vi "Close.vi"(8 "error in (no error)":errorcluster, 11 "Sequence Call Step Dict in":refnum<class "Sequence Call Step Dictionary.lvclass">) -> (0 "error out":errorcluster)   [LabVIEW 2018, in "Sequence Call Step Dictionary.lvlib" / "Sequence Call Step Dictionary.lvclass"]
uses:
  Sequence Call Step Dictionary.lvclass
  Sequence Call Step Dictionary.lvclass/Sequence Call Step Dictionary.ctl
  Controls/Sequence Call Step.ctl
  Controls/Parameter.ctl
  Private Methods/Read Database.vi
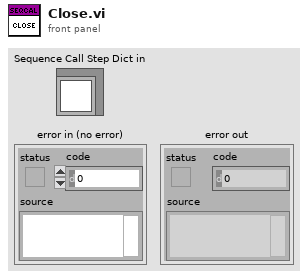
[diagram p1: front panel]
types:
  T1 = typedef "Sequence Call Step Dictionary.lvlib/Sequence Call Step Dictionary.lvclass/Sequence Call Step.ctl" = cluster{"Sequence Call Step Reference":refnum<k7>, "Sequence Call Parameters":T2[]}
  T2 = typedef "Sequence Call Step Dictionary.lvlib/Sequence Call Step Dictionary.lvclass/Parameter.ctl" = cluster{"Name":string, "PropertyObject Type":enum16{"Container", "String", "Boolean", "Number", "NamedType", "Reference", "Array", "Aperture Time"}}
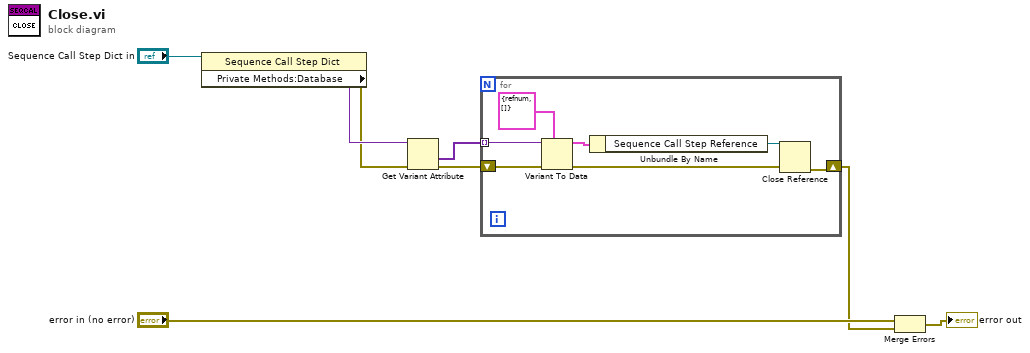
[diagram p0: block diagram]
diagram:
  n1 = property class="Sequence Call Step Dict"(reference="Sequence Call Step Dict in") -> (error out=w4:errorcluster, "Private Methods:Database"=w5:variant)  [unwired: 1 in, 1 out]
  n2 = Get Variant Attribute(Variant=w5, error in=w4) -> (values=w2:variant[], error out=w3:errorcluster)  [unwired: 2 in, 2 out]
  n3 = for {
    shift-right: [w9] -> w1
    shift-left: w3 -> [w15]
    tunnel: w2 -> [w14] mode=indexing
    n4 = Variant To Data(error in=w15, type=T1 {"Sequence Call Step Reference"=refnum, "Sequence Call Parameters"=[]} ("Cluster"), Variant=w14) -> (data=w12:T1, error out=w10:errorcluster)
    n5 = Unbundle By Name(w12) -> ("Sequence Call Step Reference"=w11:refnum<k7>)
    n6 = Close Reference(reference=w11, error in (no error)=w10) -> (error out=w9:errorcluster)
  }
  n7 = Merge Errors("error in (no error)", w1) -> (→"error out":errorcluster)
